vi "ClawUpDown.vi"(0 "Wrist":T1={"DevStatus"={"status"=FALSE, "code"=0, "source"=""}, "Pneumatics Control Module"=0, "Forward Solenoid Channel"=enum."Invalid", "Reverse Solenoid Channel"=enum."Invalid"}, 1 "Scaled Pot":dbl, 3 "State":i32, 5 "Setpoints":dbl[](array[numeric])) -> (7 "SetpointOut":i32)   [LabVIEW 2014]
uses:
  <vilib>/Rock Robotics/WPI/Solenoid/WPI_SolenoidDevRef.ctl
  <vilib>/Rock Robotics/WPI/Solenoid/WPI_SolenoidChannel.ctl
  <vilib>/Rock Robotics/WPI/Solenoid/WPI_SolenoidValue.ctl
  <vilib>/Rock Robotics/WPI/Solenoid/WPI_SolenoidSetEnum.vi
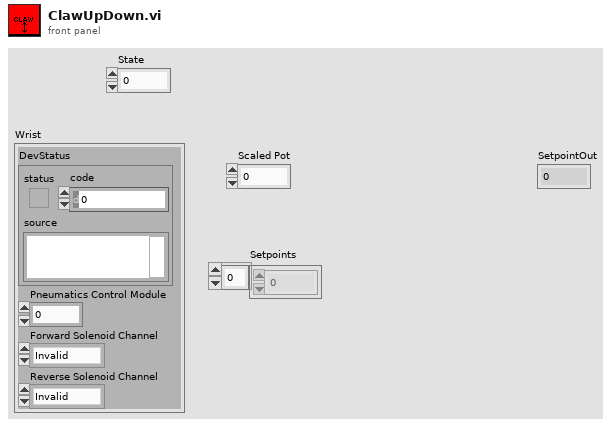
[diagram p1: front panel]
types:
  T1 = typedef "WPI_SolenoidDevRef.ctl" = cluster{"DevStatus":errorcluster, "Pneumatics Control Module":u8, "Forward Solenoid Channel":T2, "Reverse Solenoid Channel":T2}
  T2 = typedef "WPI_SolenoidChannel.ctl" = enum8{"Solenoid 0", "Solenoid 1", "Solenoid 2", "Solenoid 3", "Solenoid 4", "Solenoid 5", "Solenoid 6", "Solenoid 7", "Invalid"}
  T3 = typedef "WPI_SolenoidValue.ctl" = enum16{"Off", "On", "Forward", "Reverse"}
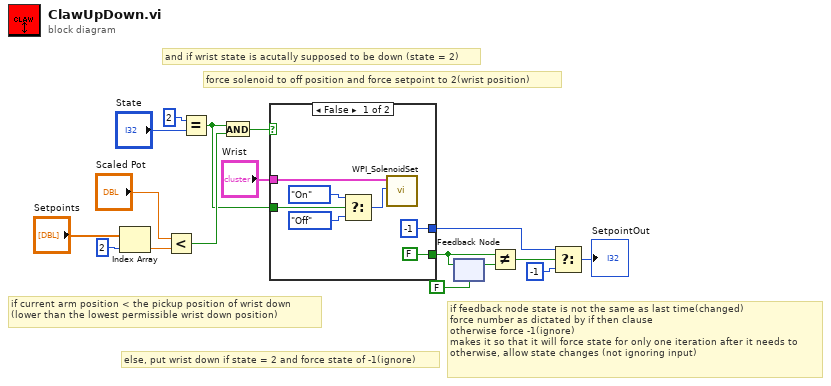
[diagram p0: block diagram]
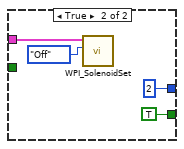
[diagram p2: hidden frame]
diagram:
  # "if feedback node state is not the same as last time(changed)\nforce number as dictated by if then clause\notherwise force -1(ignore)\nmakes it so that it will force state for only one iteration after it needs to\notherwise, allow state changes (not ignoring input)"
  # "else, put wrist down if state = 2 and force state of -1(ignore)"
  # "force solenoid to off position and force setpoint to 2(wrist position)"
  # "and if wrist state is acutally supposed to be down (state = 2)"
  # "if current arm position < the pickup position of wrist down\n(lower than the lowest permissible wrist down position)"
  n1 = Index Array(array="Setpoints", index=2) -> (element=w15:dbl)
  n2 = Less?(x="Scaled Pot", y=w15) -> (x < y?=w13:bool)
  n3 = Equal?(x=2, y="State") -> (x = y?=w8:bool)
  n4 = And(x=w8, y=w13) -> (x .and. y?=w12:bool)
  n5 = case shown="False" w12 {
    tunnel: [-1 2] -> w4
    tunnel: "Wrist" -> [w20 w27]
    tunnel: w8 -> [w19 _]
    tunnel: [FALSE TRUE] -> w6
    frame False {
      n6 = Select(t=WPI_SolenoidValue."On" ("Value"), s=w19, f=WPI_SolenoidValue."Off") -> (s? t:f=w21:T3)
      n7 = call-poly <vilib>:"WPI_SolenoidSet.vi"("Value"=w21, "SolenoidDevRef"=w20) -> ()  [unwired: 8 in, 2 out]
    }
    frame True {
      n8 = call-poly <vilib>:"WPI_SolenoidSet.vi"("Value"=WPI_SolenoidValue."Off", "SolenoidDevRef"=w27) -> ()  [unwired: 8 in, 2 out]
    }
  }
  n9 = feedback-in #1(w6) -> ()
  n10 = feedback #1(FALSE) -> (w7:bool)
  n11 = Not Equal?(x=w6, y=w7) -> (x != y?=w5:bool)
  n12 = Select(t=w4, s=w5, f=-1) -> (s? t:f=→"SetpointOut":i32)
